vi "Serialisation Type.vi"(3 "IWampMessage in":refnum<class "IWampMessage.lvclass">) -> (1 "Serialisation Type":T1)   [LabVIEW 2020, in "wamplv.lvlib" / "IWampMessage.lvclass"]
uses:
  IWampMessage.lvclass
  WAMP Client/API/TypeDefs/Serialisation.ctl
  WAMP Client/WAMP Client.lvclass
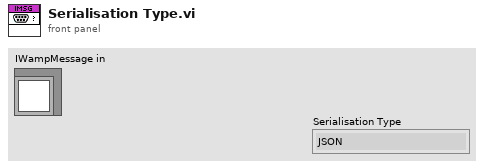
[diagram p1: front panel]
types:
  T1 = typedef "wamplv.lvlib/WAMP Client.lvclass/Serialisation.ctl" = enum16{"JSON", "MessagePack"}
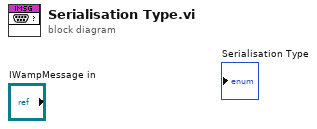
[diagram p0: block diagram]
diagram:
